vi "test.vi"   [LabVIEW 2010, in "Tank Robot.lvrbt"]
uses:
  Tank Robot.lvrbt
  <vilib>/NXT/Subs/LVHSConnector.ctl
  <vilib>/NXT/NXTIO Xnodes/AddressXNode/NXTIOAddress.xnode
  <vilib>/NXT/Subs/MotorXNode.DC Motor Type.ctl
  <vilib>/NXT/Subs/MotorXNode.2DCMotor.ctl
  <vilib>/NXT/NXTIO Xnodes/NXTIOXNode/NXTIO.xnode
  <vilib>/NXT/Dual Mode Library/prims/inRangeAndCoerce/inRangeAndCoerce_int.vi
  <vilib>/NXT/Dual Mode Library/Display/drawText.vi
  <vilib>/NXT/NXTIO Xnodes/NXTIONodeSubVIs/TETRIX IO Move DC Motors.vi
types:
  T1 = typedef "LVHSConnector.ctl" = cluster{"Hardware":string, "Flattened String":string}
  T2 = typedef "FTC ControllerState.ctl" = cluster{"Left X":i8, "Left Y":i8, "Right X":i8, "Right Y":i8, "Button Encoding 9-12":u8, "Button Encoding 1-8":u8, "POV":T3}
  T3 = typedef "FTC POVState.ctl" = i8
  T4 = typedef "MotorXNode.DC Motor Type.ctl" = enum16{"DC Motor"}
  T5 = cluster{"DC Motor":T4, "Address":i16, "Address":i16}
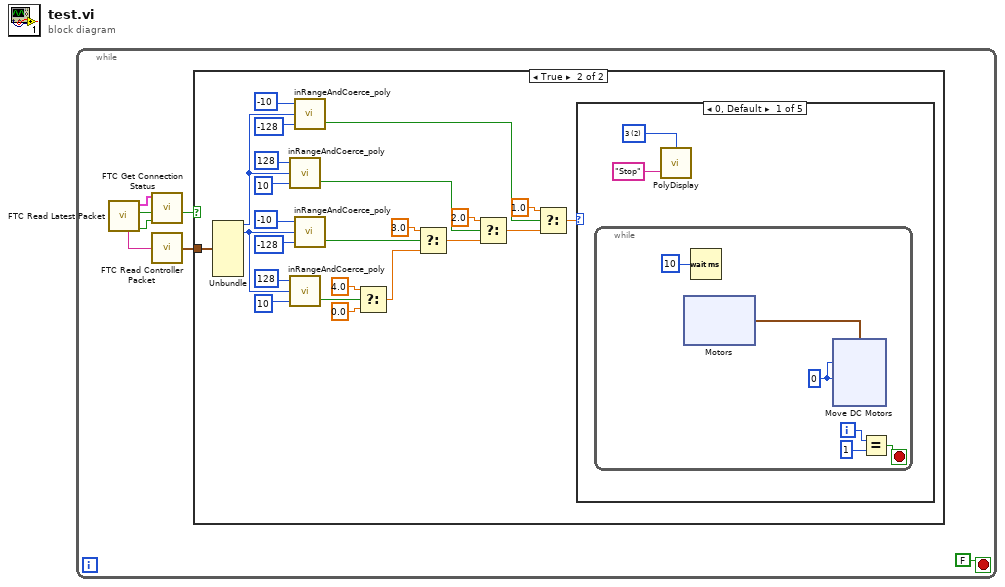
[diagram p0: block diagram]
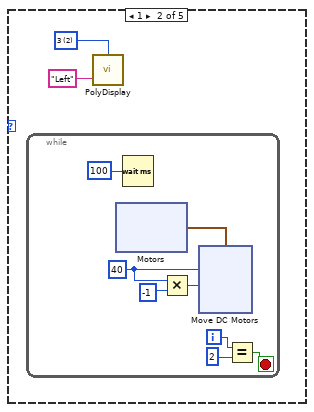
[diagram p3: hidden frame]
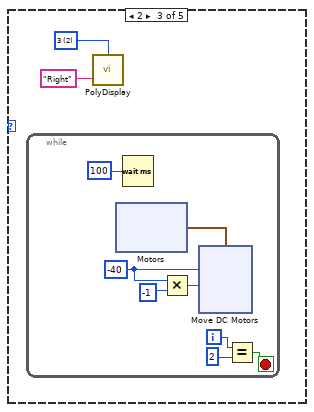
[diagram p4: hidden frame]
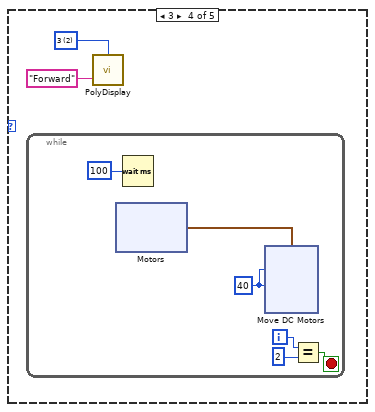
[diagram p5: hidden frame]
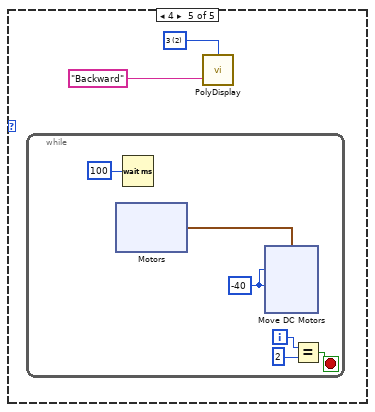
[diagram p6: hidden frame]
diagram:
  n1 = while {
    stop <- FALSE stop-if-true
    n2 = call <vilib>:"FTC Read Latest Packet.vi"() -> ("Packet Received?"=w5:bool, "Teleop?"=w6:bool, "NXT"=w4:T1, "Controller 1"=w2:string)  [unwired: 6 in, 2 out]
    n3 = call <vilib>:"FTC Get Connection Status.vi"("Packet Received?"=w5, "Stopped?"=w6, "NXT"=w4) -> ("Stopped?"=w3:bool)  [unwired: 5 in, 2 out]
    n4 = call <vilib>:"FTC Read Controller Packet.vi"("Packet"=w2) -> ("Controller State"=w1:T2)  [unwired: 4 in]
    n5 = case shown="True" w3 {
      tunnel: w1 -> [_ w31]
      frame False {
      }
      frame True {
        n6 = Unbundle(w31) -> ("Left X"=w21:i8, "Left Y"=w20:i8)  [unwired: 5 out]
        n7 = call-poly <vilib>:"inRangeAndCoerce_poly.vi"("lower limit"=10, "x"=w21, "upper limit"=128) -> ("In Range?"=w10:bool)  [unwired: 1 out]
        n8 = call-poly <vilib>:"inRangeAndCoerce_poly.vi"("lower limit"=10, "x"=w20, "upper limit"=128) -> ("In Range?"=w8:bool)  [unwired: 1 out]
        n9 = call-poly <vilib>:"inRangeAndCoerce_poly.vi"("lower limit"=-128, "x"=w21, "upper limit"=-10) -> ("In Range?"=w11:bool)  [unwired: 1 out]
        n10 = call-poly <vilib>:"inRangeAndCoerce_poly.vi"("lower limit"=-128, "x"=w20, "upper limit"=-10) -> ("In Range?"=w9:bool)  [unwired: 1 out]
        n11 = Select(t=4.0, s=w8, f=0.0) -> (s? t:f=w30:dbl)
        n12 = Select(t=3.0, s=w9, f=w30) -> (s? t:f=w29:dbl)
        n13 = Select(t=2.0, s=w10, f=w29) -> (s? t:f=w28:dbl)
        n14 = Select(t=1.0, s=w11, f=w28) -> (s? t:f=w27:dbl)
        n15 = case shown="0, Default" w27 {
          frame 0, Default {
            w32 = i16 2 items=["1", "2", "3", "4", "5", "6", "7", "8"] ("Line")
            n16 = while {
              i -> [w37]
              stop <- w34 stop-if-true
              w38 = 0
              n17 = xnode "Motors"() -> ("DC Motor"=w39:T5)
              n18 = Wait (ms)(milliseconds to wait=u32 10) -> ()  [unwired: 1 out]
              n19 = xnode "Move DC Motors"("Power/Speed 2"=w38, "Power/Speed 1"=w38, "Motors"=w39) -> ()  [unwired: 1 in, 1 out]
              n20 = Equal?(x=w37, y=1) -> (x = y?=w34:bool)
            }
            n21 = call-poly <vilib>:"PolyDisplay.vi"("Text"="Stop", "Line"=w32) -> ()  [unwired: 2 in, 1 out]
          }
          frame 1 {
            w51 = i16 2 items=["1", "2", "3", "4", "5", "6", "7", "8"] ("Line")
            n22 = while {
              i -> [w59]
              stop <- w56 stop-if-true
              w55 = 40
              n23 = xnode "Motors"() -> ("DC Motor"=w60:T5)
              n24 = Wait (ms)(milliseconds to wait=u32 100) -> ()  [unwired: 1 out]
              n25 = Multiply(x=w55, y=-1) -> (x*y=w53:i32)
              n26 = xnode "Move DC Motors"("Power/Speed 2"=w53, "Power/Speed 1"=w55, "Motors"=w60) -> ()  [unwired: 1 in, 1 out]
              n27 = Equal?(x=w59, y=2) -> (x = y?=w56:bool)
            }
            n28 = call-poly <vilib>:"PolyDisplay.vi"("Text"="Left", "Line"=w51) -> ()  [unwired: 2 in, 1 out]
          }
          frame 2 {
            w72 = i16 2 items=["1", "2", "3", "4", "5", "6", "7", "8"] ("Line")
            n29 = while {
              i -> [w80]
              stop <- w77 stop-if-true
              w76 = -40
              n30 = xnode "Motors"() -> ("DC Motor"=w81:T5)
              n31 = Wait (ms)(milliseconds to wait=u32 100) -> ()  [unwired: 1 out]
              n32 = Multiply(x=w76, y=-1) -> (x*y=w74:i32)
              n33 = xnode "Move DC Motors"("Power/Speed 2"=w74, "Power/Speed 1"=w76, "Motors"=w81) -> ()  [unwired: 1 in, 1 out]
              n34 = Equal?(x=w80, y=2) -> (x = y?=w77:bool)
            }
            n35 = call-poly <vilib>:"PolyDisplay.vi"("Text"="Right", "Line"=w72) -> ()  [unwired: 2 in, 1 out]
          }
          frame 3 {
            w93 = i16 2 items=["1", "2", "3", "4", "5", "6", "7", "8"] ("Line")
            n36 = while {
              i -> [w98]
              stop <- w95 stop-if-true
              w99 = 40
              n37 = xnode "Motors"() -> ("DC Motor"=w100:T5)
              n38 = Wait (ms)(milliseconds to wait=u32 100) -> ()  [unwired: 1 out]
              n39 = xnode "Move DC Motors"("Power/Speed 2"=w99, "Power/Speed 1"=w99, "Motors"=w100) -> ()  [unwired: 1 in, 1 out]
              n40 = Equal?(x=w98, y=2) -> (x = y?=w95:bool)
            }
            n41 = call-poly <vilib>:"PolyDisplay.vi"("Text"="Forward", "Line"=w93) -> ()  [unwired: 2 in, 1 out]
          }
          frame 4 {
            w112 = i16 2 items=["1", "2", "3", "4", "5", "6", "7", "8"] ("Line")
            n42 = while {
              i -> [w117]
              stop <- w114 stop-if-true
              w118 = -40
              n43 = xnode "Motors"() -> ("DC Motor"=w119:T5)
              n44 = Wait (ms)(milliseconds to wait=u32 100) -> ()  [unwired: 1 out]
              n45 = xnode "Move DC Motors"("Power/Speed 2"=w118, "Power/Speed 1"=w118, "Motors"=w119) -> ()  [unwired: 1 in, 1 out]
              n46 = Equal?(x=w117, y=2) -> (x = y?=w114:bool)
            }
            n47 = call-poly <vilib>:"PolyDisplay.vi"("Text"="Backward", "Line"=w112) -> ()  [unwired: 2 in, 1 out]
          }
        }
      }
    }
  }
